vi "Instrument.Command Enum to String.vi"(8 "error in (no error)":errorcluster, 10 "Commands":T1, 11 "Instrument in":refnum<class "Instrument.lvclass">) -> (0 "error out":errorcluster, 1 "Commands []":string[](array[string]), 2 "Command":string, 3 "Instrument out":refnum<class "Instrument.lvclass">)   [LabVIEW 2016, in "Instrument.lvclass"]
uses:
  Instrument.lvclass
  Typedefs/Instrument.Commands--Enum.ctl
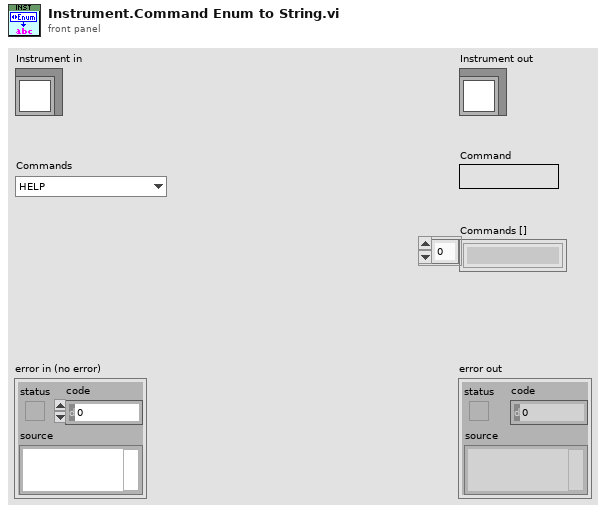
[diagram p1: front panel]
types:
  T1 = typedef "Instrument.lvclass/Instrument.Commands--Enum.ctl" = enum16{"HELP", "ACK", "getAll"}
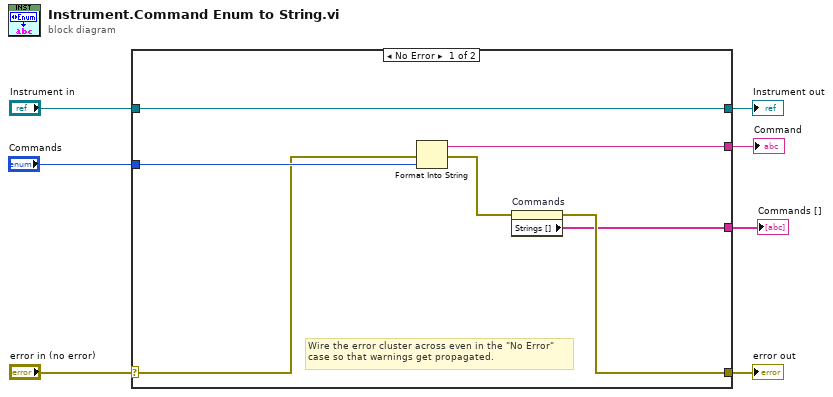
[diagram p0: block diagram]
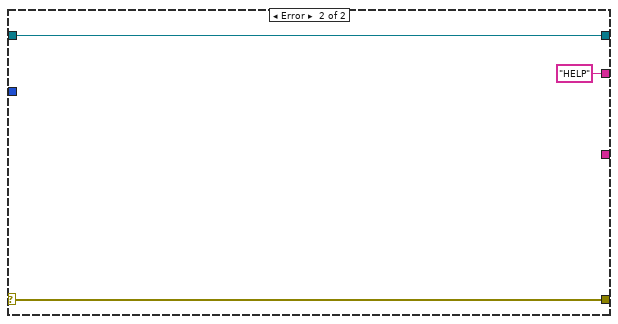
[diagram p2: hidden frame]
diagram:
  n1 = case shown="No Error" "error in (no error)" {
    selector: "error in (no error)" -> [w11 w17]
    tunnel: [w9 w17] -> w6
    tunnel: [w14 w16] -> w4
    tunnel: "Instrument in" -> [w14 w16]
    tunnel: "Commands" -> [w13 _]
    tunnel: [w12 "HELP"] -> w2
    tunnel: [w8 _] -> w1
    frame No Error {
      # "Wire the error cluster across even in the \"No Error\"\ncase so that warnings get propagated."
      n2 = Format Into String(error in=w11, w13) -> (resulting string=w12:string, error out=w10:errorcluster)  [unwired: 2 in]
      n3 = property on="Commands" class="Enum (strict)"(error in=w10) -> (error out=w9:errorcluster, "Strings []"=w8:string[])  [unwired: 1 in, 1 out]
    }
    frame Error {
    }
  }
  "error out" <- w6
  "Instrument out" <- w4
  "Command" <- w2
  "Commands []" <- w1
